vi "PC Code 1.vi"() -> ()   [LabVIEW 2014]
uses:
  <vilib>/Instr/_visa.llb/VISA Flush IO Buffer Mask.ctl
panel:
  in  "Tab Control":T1(tab)
  in  "Fish Communication Network\nVISA Port":refnum<visa-resource-name>="COM6"
  in  "GPS Network\nVISA Port":refnum<visa-resource-name>="COM8"
  in  "Fish Communication Network\nError In":errorcluster
  in  "GPS Network\nError In":errorcluster
  out "GPS Network \nHandshake Successful?":bool
  out "Comms Network \nHandshake Successful?":bool
  out "Handshake Complete":bool
  out "Handshake Aborted":bool
  in  "Comms Input 1":string="World"
  in  "Comms Input 2":string="Hello"
  out "Currently Transmitting\nComms Input":string
  in  "GPS Input 1":string="Hello"
  in  "GPS Input 2":string="World"
  out "Currently Transmitting \nGPS Input":string
  out "Running?":bool
  in  "stop":bool caption="ESTOP"
  out "error out":errorcluster
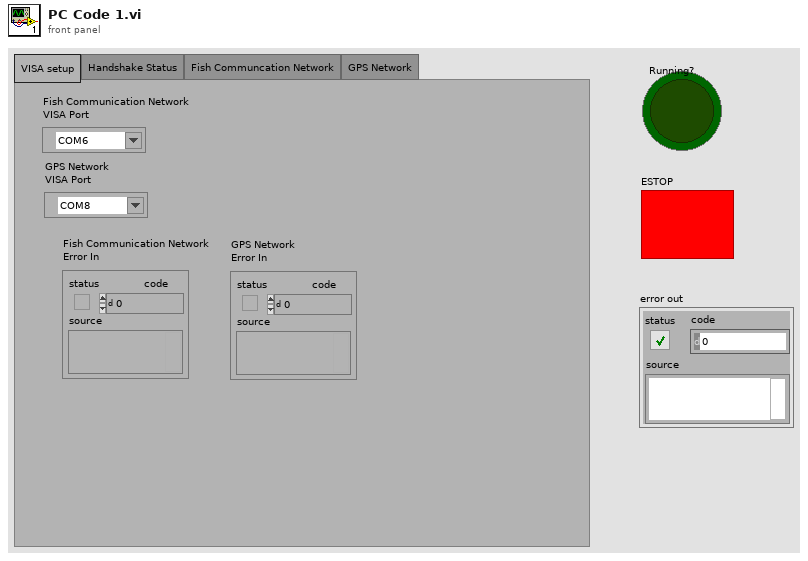
[diagram p1: front panel]
types:
  T1 = enum32{"VISA setup", "Handshake Status", "Fish Communcation Network", "GPS Network"}
  T2 = typedef "VISA Flush IO Buffer Mask.ctl" = u16
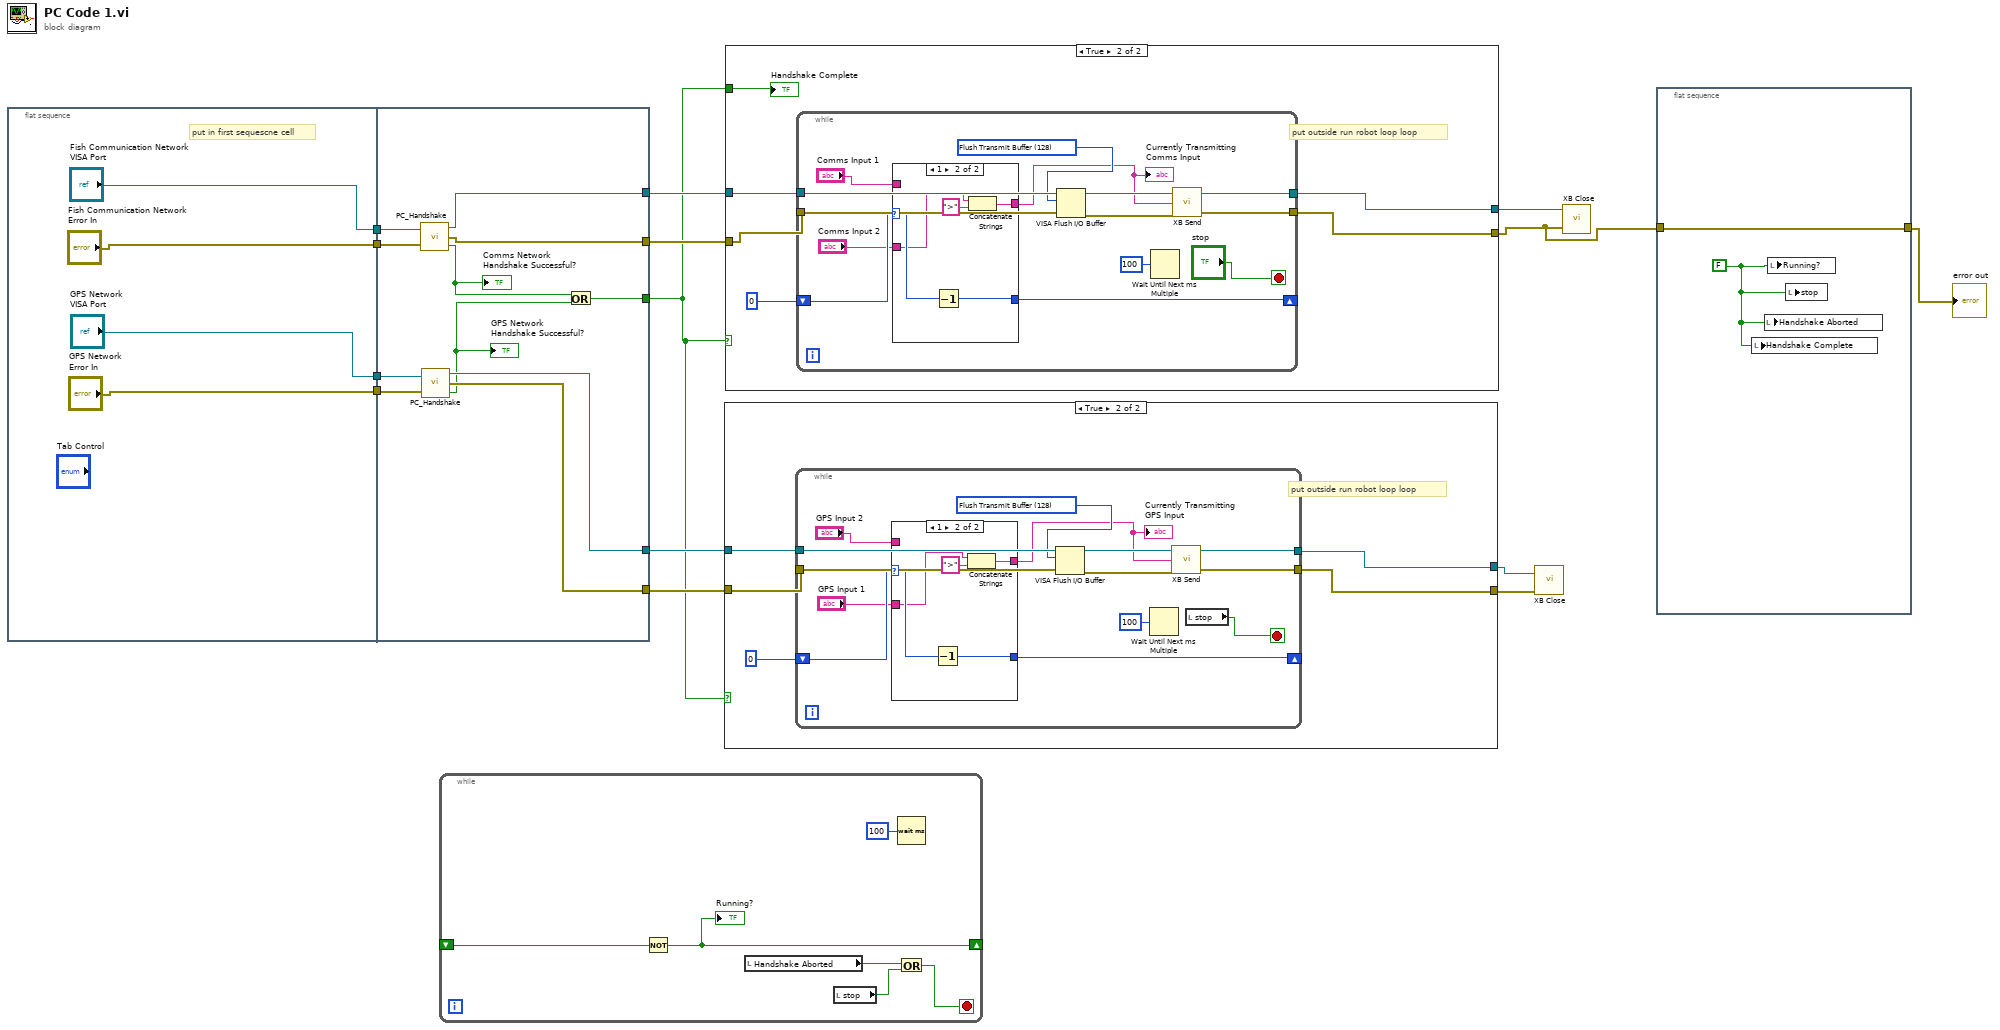
[diagram p0: block diagram]
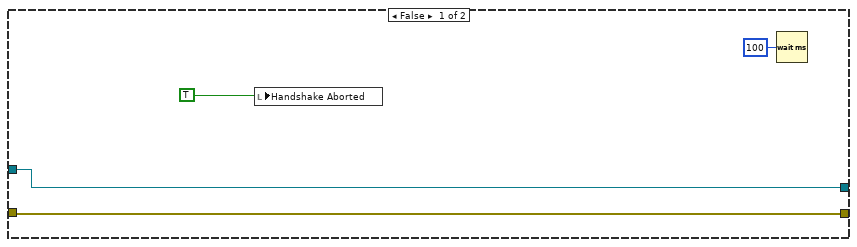
[diagram p2: hidden frame]
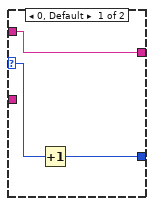
[diagram p3: hidden frame]
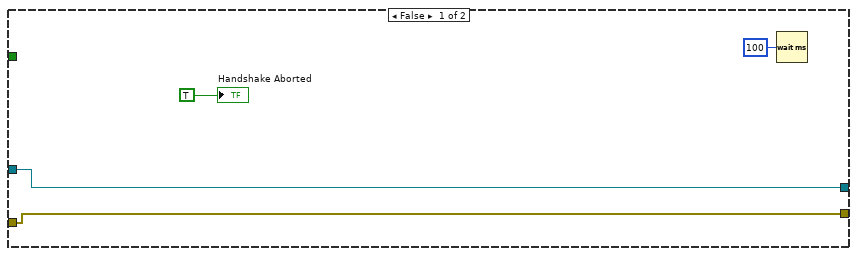
[diagram p4: hidden frame]
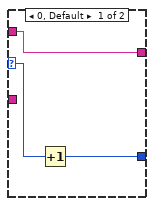
[diagram p5: hidden frame]
diagram:
  n1 = flat-sequence {
    tunnel: ["Fish Communication Network\nVISA Port"] -> w9
    tunnel: ["Fish Communication Network\nError In"] -> w8
    tunnel: ["GPS Network\nVISA Port"] -> w7
    tunnel: ["GPS Network\nError In"] -> w6
    tunnel: w9 -> [w29]
    tunnel: w8 -> [w28]
    tunnel: w7 -> [w27]
    tunnel: w6 -> [w26]
    tunnel: [w25] -> w5
    tunnel: [w24] -> w4
    tunnel: [w23] -> w3
    tunnel: [w22] -> w2
    tunnel: [w21] -> w1
    frame #0 {
      # "put in first sequescne cell"
    }
    frame #1 {
      n2 = call "PC_Handshake.vi"("VISA resource name"=w29, "error in"=w28) -> ("VISA resource name out"=w25:refnum<visa-resource-name>, "error out"=w24:errorcluster, "Handshake Successful?"=w19:bool)
      "Comms Network \nHandshake Successful?" <- w19
      n3 = call "PC_Handshake.vi"("VISA resource name"=w27, "error in"=w26) -> ("VISA resource name out"=w23:refnum<visa-resource-name>, "error out"=w22:errorcluster, "Handshake Successful?"=w20:bool)
      "GPS Network \nHandshake Successful?" <- w20
      n4 = Or(x=w19, y=w20) -> (x .or. y?=w21:bool)
    }
  }
  n5 = while {
    shift-right: [w34] -> _
    shift-left: _ -> [w35]
    stop <- w32 stop-if-true
    n6 = Not(x=w35) -> (.not. x?=w34:bool)
    "Running?" <- w34
    n7 = local read "Handshake Aborted"() -> (w30:bool)
    n8 = local read "stop"() -> (w31:bool)
    n9 = Wait (ms)(milliseconds to wait=u32 100) -> ()  [unwired: 1 out]
    n10 = Or(x=w30, y=w31) -> (x .or. y?=w32:bool)
  }
  n11 = case shown="True" w1 {
    tunnel: w3 -> [w38 w44]
    tunnel: w2 -> [w37 w43]
    tunnel: [w38 w41] -> w12
    tunnel: [w37 w40] -> w11
    frame False {
      n12 = local write "Handshake Aborted"(TRUE) -> ()
      n13 = Wait (ms)(milliseconds to wait=u32 100) -> ()  [unwired: 1 out]
    }
    frame True {
      # "put outside run robot loop loop"
      n14 = while {
        tunnel: w44 -> [w55]
        tunnel: w43 -> [w53]
        tunnel: [w56] -> w40
        tunnel: [w57] -> w41
        shift-right: [w49] -> _
        shift-left: 0 -> [w50]
        stop <- w45 stop-if-true
        w51 = T2 128 items=["Flush Receive Buffer"=16, "Write Transmit Buffer to Device"=32, "Flush Receive Buffer (No I/O)"=64, "Flush Transmit Buffer"=128] ("Mask")
        n15 = case shown="1" w50 {
          selector: w50 -> [w61 w65]
          tunnel: [w60 w66] -> w49
          tunnel: "GPS Input 1" -> [_ w63]
          tunnel: "GPS Input 2" -> [w59 _]
          tunnel: [w59 w62] -> w46
          frame 0, Default {
            n16 = Increment(x=w61) -> (x+1=w60:i32)
          }
          frame 1 {
            n17 = Decrement(x=w65) -> (x-1=w66:i32)
            n18 = Concatenate Strings(w63, ">" ("string")) -> (w62:string)
          }
        }
        "Currently Transmitting \nGPS Input" <- w46
        n19 = VISA Flush I/O Buffer(VISA resource name=w55, mask (16)=w51, error in (no error)=w53) -> (VISA resource name out=w54:refnum<visa-resource-name>, error out=w52:errorcluster)
        n20 = Wait Until Next ms Multiple(millisecond multiple=u32 100) -> ()  [unwired: 1 out]
        n21 = call "XB Send.vi"("error in (no error)"=w52, "String"=w46, "VISA resource name"=w54) -> ("error out"=w56:errorcluster, "VISA resource name out"=w57:refnum<visa-resource-name>)  [unwired: 1 out]
        n22 = local read "stop"() -> (w45:bool)
      }
    }
  }
  n23 = case shown="True" w1 {
    tunnel: w5 -> [w68 w76]
    tunnel: w1 -> [_ w72]
    tunnel: [w68 w74] -> w14
    tunnel: [w67 w73] -> w10
    tunnel: w4 -> [w67 w71]
    frame False {
      n24 = Wait (ms)(milliseconds to wait=u32 100) -> ()  [unwired: 1 out]
      "Handshake Aborted" <- TRUE
    }
    frame True {
      # "put outside run robot loop loop"
      n25 = while {
        tunnel: w76 -> [w86]
        tunnel: w71 -> [w84]
        tunnel: [w87] -> w73
        tunnel: [w88] -> w74
        shift-right: [w80] -> _
        shift-left: 0 -> [w81]
        stop <- "stop" stop-if-true
        w82 = T2 128 items=["Flush Receive Buffer"=16, "Write Transmit Buffer to Device"=32, "Flush Receive Buffer (No I/O)"=64, "Flush Transmit Buffer"=128] ("Mask")
        n26 = case shown="1" w81 {
          selector: w81 -> [w93 w97]
          tunnel: [w92 w98] -> w80
          tunnel: "Comms Input 2" -> [_ w95]
          tunnel: "Comms Input 1" -> [w91 _]
          tunnel: [w91 w94] -> w77
          frame 0, Default {
            n27 = Increment(x=w93) -> (x+1=w92:i32)
          }
          frame 1 {
            n28 = Decrement(x=w97) -> (x-1=w98:i32)
            n29 = Concatenate Strings(w95, ">" ("string")) -> (w94:string)
          }
        }
        "Currently Transmitting\nComms Input" <- w77
        n30 = VISA Flush I/O Buffer(VISA resource name=w86, mask (16)=w82, error in (no error)=w84) -> (VISA resource name out=w85:refnum<visa-resource-name>, error out=w83:errorcluster)
        n31 = Wait Until Next ms Multiple(millisecond multiple=u32 100) -> ()  [unwired: 1 out]
        n32 = call "XB Send.vi"("error in (no error)"=w83, "String"=w77, "VISA resource name"=w85) -> ("error out"=w87:errorcluster, "VISA resource name out"=w88:refnum<visa-resource-name>)  [unwired: 1 out]
      }
      "Handshake Complete" <- w72
    }
  }
  n33 = call "XB Close.vi"("error in (no error)"=w11, "VISA resource name"=w12) -> ()
  n34 = call "XB Close.vi"("error in (no error)"=w10, "VISA resource name"=w14) -> ()
  n35 = flat-sequence {
    tunnel: w10 -> [w99]
    tunnel: [w99] -> w13
    frame #0 {
      w100 = FALSE
      n36 = local write "Handshake Complete"(w100) -> ()
      n37 = local write "Handshake Aborted"(w100) -> ()
      n38 = local write "Running?"(w100) -> ()
      n39 = local write "stop"(w100) -> ()
    }
  }
  "error out" <- w13
